vi "GlobalSettings.vi"() -> ()   [LabVIEW 2011]
uses:
  mirror/E517_Controller_names.ctl
  mirror/E517_Termination_character.ctl
  mirror/E517_Available_interfaces.ctl
  mirror/E517_Available_DLL_interfaces.ctl
  mirror/E517_Available_DLLs.ctl
panel:
  out "scanner global out":T6 {"Main-Global-Config out"."Global-Config"."DLL Interface\nConfiguration"."DLL for Device" items=["C-843", "C-844", "E-710", "C-843.PM", "C-865", "E-761", "Mercury", "E-755", "E-753", "C-866", "E-712", "E-725", "E-861", "C-867", "E-517"]; "Main-Global-Config out"."Global-Config"."DLL Interface\nConfiguration"."DLL Interface" items=["RS232", "GPIB", "Board", "TCP-IP", "USB", "RS232_DC"]; "Main-Global-Config out"."Global-Config"."Interface configuration"."Interface" items=["RS232", "GPIB", "DLL", "TCP-IP", "USB", "Analog"]}
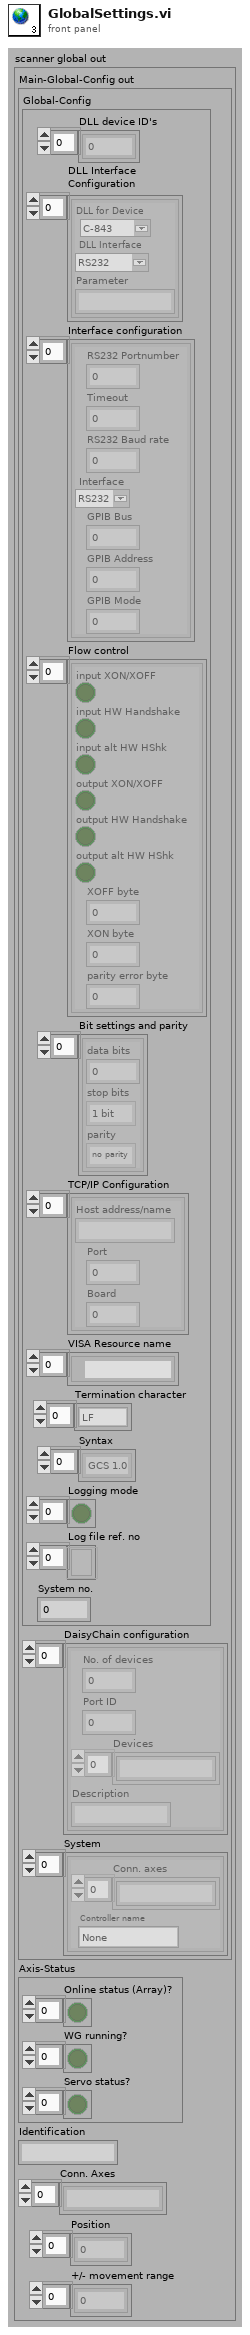
[diagram p1: front panel]
types:
  T1 = typedef "E517_Available_DLLs.ctl" = u16
  T2 = typedef "E517_Available_DLL_interfaces.ctl" = u16
  T3 = typedef "E517_Available_interfaces.ctl" = u16
  T4 = typedef "E517_Termination_character.ctl" = enum16{"LF", "CR", "LFCR", "CRLF"}
  T5 = typedef "E517_Controller_names.ctl" = enum16{"None", "Analog", "C-702", "C-843", "C-843.PM", "C-844", "C-848", "C-865", "C-866", "C-867", "C-880", "E-516", "E-517", "E-710", "E-712", "E-725", "E-753", "E-755", "E-761", "E-816", "E-861", "F-206", "M-840", "M-850", "M-8X0", "Mercury"}
  T6 = cluster{"Main-Global-Config out":cluster{"Global-Config":cluster{"DLL device ID's":i32[], "DLL Interface\nConfiguration":cluster{"DLL for Device":T1, "DLL Interface":T2, "Parameter":string}[], "Interface configuration":cluster{"RS232 Portnumber":i32, "Timeout":i32, "RS232 Baud rate":u32, "Interface":T3, "GPIB Bus":i32, "GPIB Address":i32, "GPIB Mode":i32}[], "Flow control":cluster{"input XON/XOFF":bool, "input HW Handshake":bool, "input alt HW HShk":bool, "output XON/XOFF":bool, "output HW Handshake":bool, "output alt HW HShk":bool, "XOFF byte ":u8, "XON byte":u8, "parity error byte":u16}[], "Bit settings and parity":cluster{"data bits":u16, "stop bits":enum16{"1 bit", "1.5 bits", "2 bits"}, "parity":enum16{"no parity", "odd parity", "even parity", "mark parity", "space parity"}}[], "TCP/IP Configuration":cluster{"Host address/name":string, "Port":i32, "Board":i32}[], "VISA Resource name":refnum<visa-resource-name>[], "Termination character":T4[], "Syntax":enum16{"GCS 1.0", "GCS 2.0"}[], "Logging mode":bool[], "Log file ref. no":refnum<file>[], "System no.":i32}, "DaisyChain configuration":cluster{"No. of devices":i32, "Port ID":i32, "Devices":string[], "Description":string}[], "System":cluster{"Conn. axes":string[], "Controller name":T5}[]}, "Axis-Status":cluster{"Online status (Array)?":bool[], "WG running?":bool[], "Servo status?":bool[]}, "Identification":string, "Conn. Axes":string[], "Position":dbl[], "+/- movement range":dbl[]}
diagram:
